vi "Test PLL.vi"(8 "error in (no error)":errorcluster, 11 "Lockin.DAQ":refnum<class "Instrument.DAQ.lvclass">) -> (0 "error out":errorcluster, 3 "Lockin.DAQ out":refnum<class "Instrument.DAQ.lvclass">)   [LabVIEW 2019, in "Instrument.Lockin.lvlib" / "Instrument.DAQ.lvclass"]
uses:
  Instrument.DAQ.lvclass
  DAQmx/DAQmx.lvclass
  Instrument.Lockin/Typedefs/Results Type--Enum.ctl
  Instrument.Lockin/Instrument.Lockin.lvclass
  Typedefs/DeviceInfo--Cluster.ctl
  C:/Program Files/National Instruments/LabVIEW 2019/vi.lib/JKI/JKI SMO/SMO/SMO.lvclass
  Typedefs/DAQ.Sampling.Sampling--Cluster.ctl
  Typedefs/AO.Channel.Function--Enum.ctl
  Typedefs/AO.Channel--Cluster.ctl
  Typedefs/AO.Channel--Cluster--Array.ctl
  Typedefs/REF.Channel--Cluster.ctl
  Typedefs/REF.Channel--Cluster--Array.ctl
  Typedefs/AI.Channel--Cluster.ctl
  Typedefs/AI.Channel--Cluster--Array.ctl
panel:
  in  "Step?":bool
  in  "time (ms)":u32=5000
  out "Numeric":i32
  out "loop time":dbl format="%#_6p"
  out "Y Chart":dbl[](graph)
  out "X Chart":dbl[](graph)
  out "Frequency Chart":dbl[](graph)
  in  "Configuration.AI Channels":T1=[{"Enable?"=TRUE, "Channel"=1, "References"=[1], "reference index"=0}] {"reference index" min=1; "References" items=["", "1", "2", "3", "4", "5", "6", "7", "8", "9"]; "Channel" min=1}
  in  "Configuration.Channels: REF":T3=[{"Enable?"=TRUE, "Channel"=1, "Frequency"=13.0, "Phase"=0.0, "TC"=0.1, "Roll-Off"=2}] {"Roll-Off" min=1 max=4; "TC" min=1e-06 max=100.0 format="%#_3p"; "Phase" format="%#_3p"; "Frequency" min=1e-06 max=102400.0 format="%#_6p"; "Channel" min=1}
  in  "Channels: AO":T5=[{"Enable?"=TRUE, "Channel"=1, "Amplitude"=0.001, "Offset"=0.0, "Frequency"=13.0, "Phase"=0.0, "Function"=enum."sine", "Sweeping?"=FALSE, "Limit AC"=FALSE, "Limit DC?"=FALSE, "Duty Cycle"=FALSE}] {"Phase" format="%#_3g"; "Frequency" min=0.0001 max=200000.0 format="%#_6p"; "Offset" format="%#_6p"; "Amplitude" min=0.0 max=10.0 format="%#_6p"}
  out "Phase Chart":dbl[](graph)
  out "Waveform Graph":waveform(dbl)[](graph)=[{"t0"=timestamp(0 s since 1904-01-01), "dt"=1.0, "Y"=[]}, {"t0"=timestamp(0 s since 1904-01-01), "dt"=1.0, "Y"=[]}]
  in  "sampling":T8={"Fs"=204789.0, "#s"=15753} {"Fs" format="%#_13g"}
  in  "stop":bool
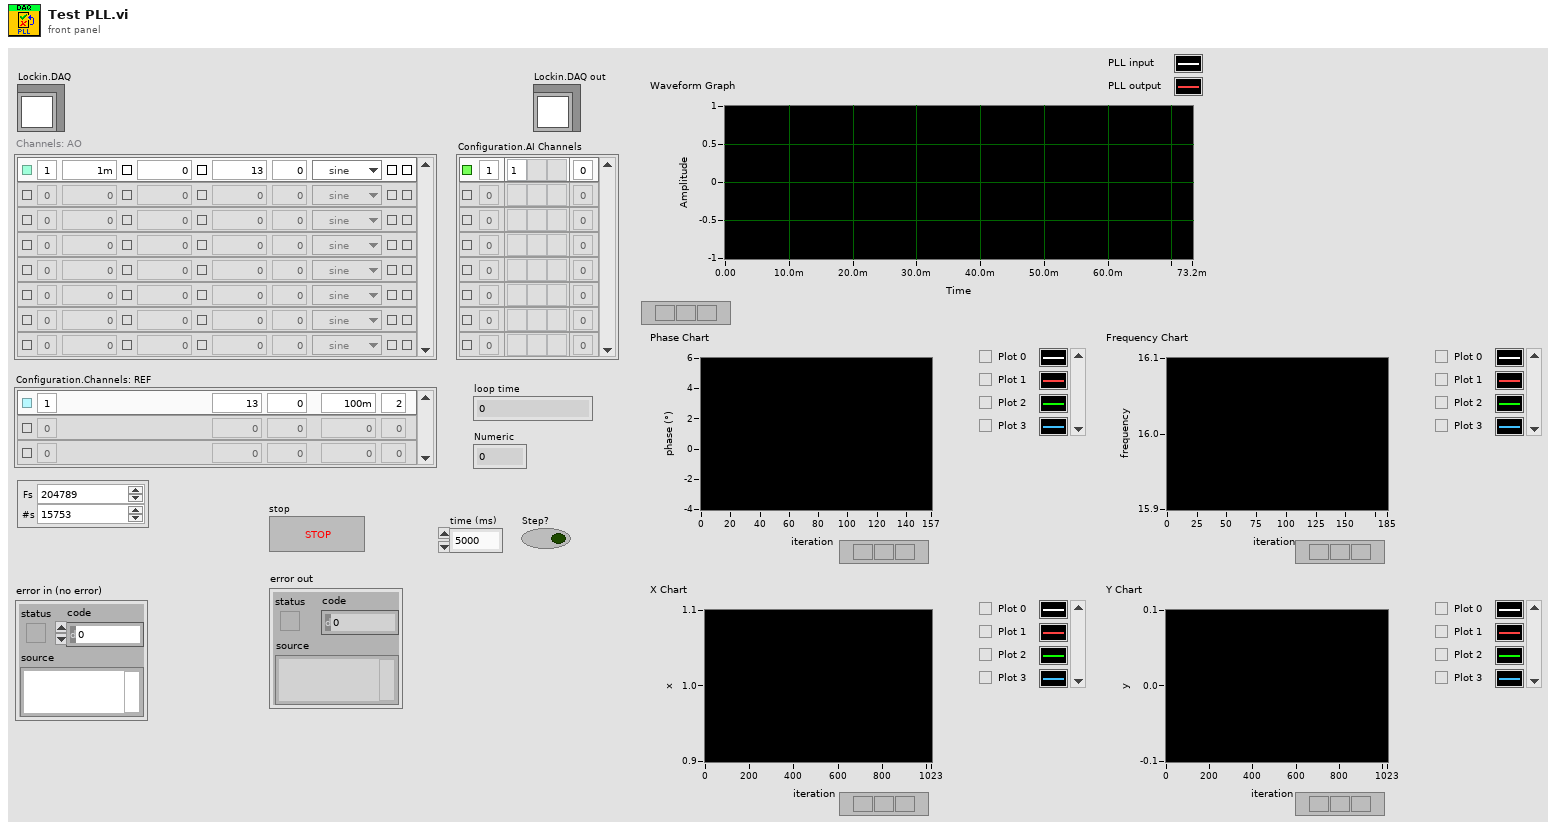
[diagram p1: front panel]
types:
  T1 = typedef "Instrument.Lockin.lvlib/Instrument.DAQ.lvclass/AI.Channel--Cluster--Array.ctl" = T2[]
  T2 = typedef "Instrument.Lockin.lvlib/Instrument.DAQ.lvclass/AI.Channel--Cluster.ctl" = cluster{"Enable?":bool, "Channel":i32, "References":u16[], "reference index":i32}
  T3 = typedef "Instrument.Lockin.lvlib/Instrument.DAQ.lvclass/REF.Channel--Cluster--Array.ctl" = T4[]
  T4 = typedef "Instrument.Lockin.lvlib/Instrument.DAQ.lvclass/REF.Channel--Cluster.ctl" = cluster{"Enable?":bool, "Channel":i32, "Frequency":dbl, "Phase":dbl, "TC":dbl, "Roll-Off":i32}
  T5 = typedef "Instrument.Lockin.lvlib/Instrument.DAQ.lvclass/AO.Channel--Cluster--Array.ctl" = T6[]
  T6 = typedef "Instrument.Lockin.lvlib/Instrument.DAQ.lvclass/AO.Channel--Cluster.ctl" = cluster{"Enable?":bool, "Channel":i32, "Amplitude":dbl, "Offset":dbl, "Frequency":dbl, "Phase":dbl, "Function":T7, "Sweeping?":bool, "Limit AC":bool, "Limit DC?":bool, "Duty Cycle":bool}
  T7 = typedef "Instrument.Lockin.lvlib/Instrument.DAQ.lvclass/AO.Channel.Function--Enum.ctl" = enum16{"sine", "square", "triangle", "saw"}
  T8 = typedef "Instrument.Lockin.lvlib/Instrument.DAQ.lvclass/DAQ.Sampling.Sampling--Cluster.ctl" = cluster{"Fs":dbl, "#s":i32}
  T9 = typedef "Instrument.Lockin.lvlib/Instrument.DAQ.lvclass/DeviceInfo--Cluster.ctl" = cluster{"DeviceName":string, "DevIsSimulated":bool, "DeviceSerialNumber":string, "ProductType":string, "ProductCategory":i32, "ProductNumber":u32, "ChassisNumber":u32, "SlotNumber":u32, "ChassisName":string, "ChassisSerialNumber":string, "DevTemp":dbl, "SelfCal.LastDate/Time":string, "SelfCal.LastTemp":dbl, "calibration due?":bool}
  T10 = typedef "Instrument.Lockin.lvlib/Instrument.Lockin.lvclass/Results Type--Enum.ctl" = enum16{"X", "Y", "R", "Theta", "Mean"}
  T11 = typedef "Instrument.Lockin.lvlib/Instrument.DAQ.lvclass/Results--Cluster.ctl" = cluster{"Time Stamp":timestamp, "Results (Dictionary)":cluster{"key":string, "value":dbl[]}[]}
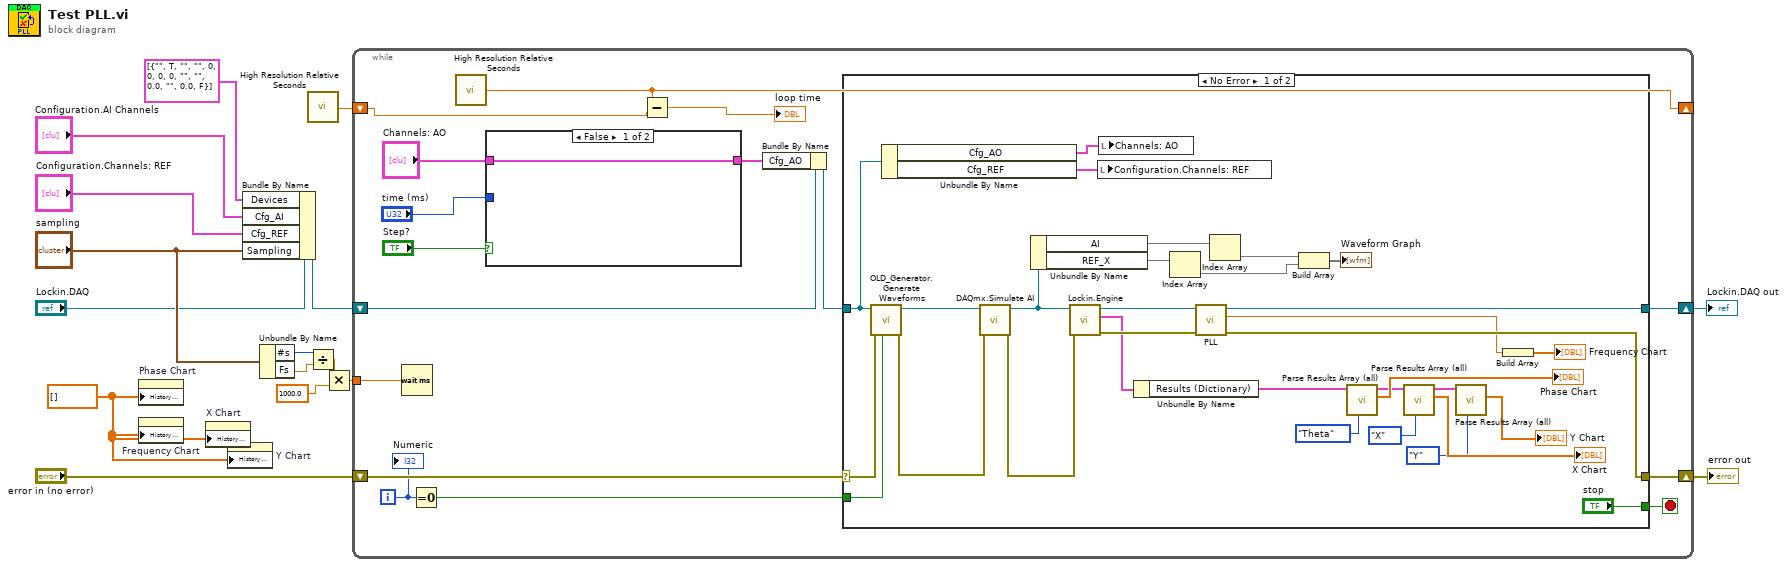
[diagram p0: block diagram]
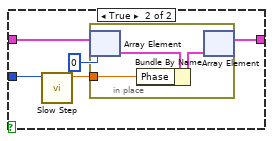
[diagram p2: hidden frame]
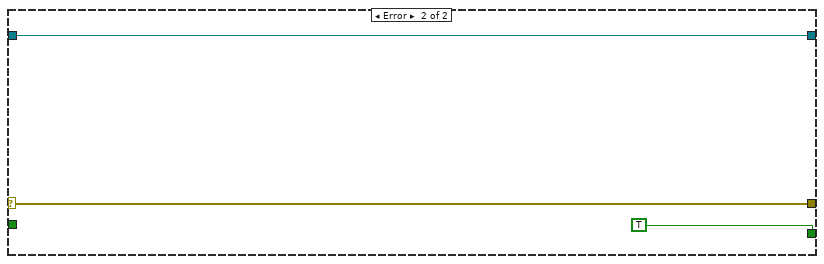
[diagram p3: hidden frame]
diagram:
  w1 = dbl[] [] ("History Data")
  n1 = property on="Phase Chart" class="WFChart (strict)"("History Data"=w1) -> ()  [unwired: 2 in, 2 out]
  n2 = property on="Frequency Chart" class="WFChart (strict)"("History Data"=w1) -> ()  [unwired: 2 in, 2 out]
  n3 = property on="X Chart" class="WFChart (strict)"("History Data"=w1) -> ()  [unwired: 2 in, 2 out]
  n4 = property on="Y Chart" class="WFChart (strict)"("History Data"=w1) -> ()  [unwired: 2 in, 2 out]
  n5 = Bundle By Name(cluster="Lockin.DAQ", "Devices"=T9[] [{"DeviceName"="", "DevIsSimulated"=TRUE, "DeviceSerialNumber"="", "ProductType"="", "ProductCategory"=0, "ProductNumber"=0, "ChassisNumber"=0, "SlotNumber"=0, "ChassisName"="", "ChassisSerialNumber"="", "DevTemp"=0.0, "SelfCal.LastDate/Time"="", "SelfCal.LastTemp"=0.0, "calibration due?"=FALSE}] ("Configuration.DAQ.Devices"), "Cfg_AI"="Configuration.AI Channels", "Cfg_REF"="Configuration.Channels: REF", "Sampling"="sampling") -> (w6:refnum<class "Instrument.DAQ.lvclass">)
  n6 = Unbundle By Name("sampling") -> ("#s"=w8:i32, "Fs"=w9:dbl)
  n7 = call <vilib>:"High Resolution Relative Seconds.vi"() -> ("relative seconds"=w2:dbl)
  n8 = Divide(x=w8, y=w9) -> (x/y=w10:dbl)
  n9 = Multiply(x=w10, y=1000.0) -> (x*y=w5:dbl)
  n10 = while {
    shift-right: [w31] -> w15
    shift-left: "error in (no error)" -> [w32]
    shift-right: [w30] -> w14
    shift-left: w6 -> [w25]
    tunnel: w5 -> [w26]
    shift-right: [w22] -> _
    shift-left: w2 -> [w23]
    i -> [w28]
    stop <- w27 stop-if-true
    n11 = Wait (ms)(milliseconds to wait=w26) -> ()  [unwired: 1 out]
    n12 = Equal To 0?(x=w28) -> (x = 0?=w29:bool)
    n13 = call <vilib>:"High Resolution Relative Seconds.vi"() -> ("relative seconds"=w22:dbl)
    n14 = case shown="False" "Step?" {
      tunnel: "Channels: AO" -> [w33 w38]
      tunnel: [w33 w36] -> w19
      tunnel: "time (ms)" -> [_ w34]
      frame False {
      }
      frame True {
        n15 = call "Slow Step.vi"("time (ms)"=w34) -> ("f"=w35:dbl)  [unwired: 10 in]
        n16 = in-place {
          in-place-border: w35 -> [w39]
          n17 = in-place-array #1(w38, 0) -> (w41:T6)
          n18 = Bundle By Name(cluster=w41, "Phase"=w39) -> (w40:T6)
          n19 = in-place-array #1(w40) -> (w36:T5)  [unwired: 1 out]
        }
      }
    }
    n20 = Subtract(x=w22, y=w23) -> (x-y=→"loop time":dbl)
    n21 = Bundle By Name(cluster=w25, "Cfg_AO"=w19) -> (w24:refnum<class "Instrument.DAQ.lvclass">)
    n22 = case shown="No Error" w32 {
      selector: w32 -> [w68 w75]
      tunnel: [w63 w75] -> w31
      tunnel: [w45 w74] -> w30
      tunnel: w24 -> [w61 w74]
      tunnel: w29 -> [w67 _]
      tunnel: ["stop" TRUE ("stop")] -> w27
      frame No Error {
        n23 = call "OLD_Generator.Generate Waveforms.vi"("reset phase?"=w67, "error in (no error)"=w68, "Instrument.DAQ"=w61) -> ("error out"=w42:errorcluster, "Instrument.DAQ"=w70:refnum<class "Instrument.DAQ.lvclass">)  [unwired: 6 in, 1 out]
        n24 = Unbundle By Name(w61) -> ("Cfg_AO"=w54:T5, "Cfg_REF"=w60:T3)
        n25 = call "DAQmx.Simulate AI.vi"("error in (no error)"=w42, "DAQmx in"=w70) -> ("error out"=w64:errorcluster, "DAQmx out"=w66:refnum<class "DAQmx.lvclass">)  [unwired: 6 in, 2 out]
        n26 = Unbundle By Name(w66) -> ("AI"=w69, "REF_X"=w59)
        n27 = call "Lockin.Engine.vi"("error in (no error)"=w64, "Instrument.DAQ"=w66) -> ("error out"=w65:errorcluster, "Results (X,Y,R,Theta,Mean)"=w62:T11, "Instrument.DAQ out"=w47:refnum<class "Instrument.DAQ.lvclass">)  [unwired: 5 in, 2 out]
        n28 = local write "Configuration.Channels: REF"(w60) -> ()
        n29 = local write "Channels: AO"(w54) -> ()
        n30 = Unbundle By Name(w62) -> ("Results (Dictionary)"=w52:cluster{"key":string, "value":dbl[]}[])
        n31 = Index Array(array=w59) -> (element=w43)  [unwired: 1 in]
        n32 = call "PLL.vi"("error in (no error)"=w65, "Instrument.DAQ in"=w47) -> ("error out"=w63:errorcluster, "frequency out"=w46:dbl, "Instrument.DAQ out"=w45:refnum<class "Instrument.DAQ.lvclass">)  [unwired: 6 in, 1 out]
        n33 = Index Array(array=w69) -> (element=w44)  [unwired: 1 in]
        n34 = Build Array(w44, w43) -> (→"Waveform Graph":void[])
        n35 = call "Parse Results Array (all).vi"("Type"=Results_Type--Enum."Theta", "Results (Dictionary)"=w52) -> ("Data"=→"Phase Chart":dbl[], "Results (Dictionary)"=w51:cluster{"key":string, "value":dbl[]}[])  [unwired: 6 in, 2 out]
        n36 = call "Parse Results Array (all).vi"("Type"=Results_Type--Enum."X", "Results (Dictionary)"=w51) -> ("Data"=→"X Chart":dbl[], "Results (Dictionary)"=w50:cluster{"key":string, "value":dbl[]}[])  [unwired: 6 in, 2 out]
        n37 = call "Parse Results Array (all).vi"("Type"=Results_Type--Enum."Y", "Results (Dictionary)"=w50) -> ("Data"=→"Y Chart":dbl[])  [unwired: 6 in, 3 out]
        n38 = Build Array(w46) -> (→"Frequency Chart":dbl[])
      }
      frame Error {
      }
    }
    "Numeric" <- w28
  }
  "error out" <- w15
  "Lockin.DAQ out" <- w14
